vi "Calc Resistive Voltage.vi"(8 "Alpha":fxp<+/-,34,10>, 9 "T inlet":T1 format="%_6g", 10 "Current":T1 format="%_6g", 11 "Coil Coefficients":fxp<+/-,38,12>[](array[numeric])=[0.0, 0.0, 0.0]) -> (2 "Resistance":T1 format="%_6g", 3 "Voltage":T1 format="%_6g")   [LabVIEW 2017]
doc: "Author: Scott Hannahs <sth@magnet.fsu.edu>\nCopyright 2018 Florida State University, All rights reserved."
uses:
  SCH Data Controls/SCH Data 2 RT.ctl
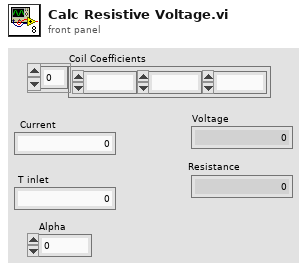
[diagram p1: front panel]
types:
  T1 = typedef "SCH Data 2 RT.ctl" = fxp<+/-,38,12>
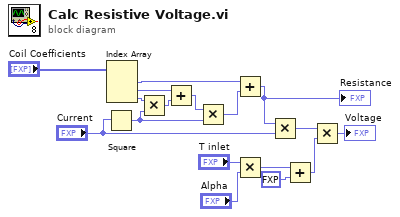
[diagram p0: block diagram]
diagram:
  n1 = Square(x="Current") -> (x^2=w11:fxp<+,38,12>)
  n2 = Index Array(array="Coil Coefficients") -> (element #1=w13:fxp<+/-,38,12>, element #2=w9:fxp<+/-,38,12>, element #3=w7:fxp<+/-,38,12>)  [unwired: 3 in]
  n3 = Multiply(x=w7, y=w11) -> (x*y=w8:fxp<+/-,38,12>)
  n4 = Add(x=w9, y=w8) -> (x+y=w10:fxp<+/-,38,12>)
  n5 = Multiply(x=w10, y=w11) -> (x*y=w12:fxp<+/-,38,12>)
  n6 = Add(x=w13, y=w12) -> (x+y=w14:fxp<+/-,38,12>)
  "Resistance" <- w14
  n7 = Multiply(x="T inlet", y="Alpha") -> (x*y=w3:T1)
  n8 = Multiply(x=w14, y="Current") -> (x*y=w16:T1)
  n9 = Add(x=w3, y=fxp<+/-,38,12> 1.0) -> (x+y=w1:T1)
  n10 = Multiply(x=w16, y=w1) -> (x*y=→"Voltage":T1)
